vi "ADAM_Hi-Tec_convert.vi"(0 "Ch Name":string, 1 "Raw":dbl format="%.3f", 3 "Channel Read":string) -> (5 "Q release (l/min)":dbl format="%.2f", 6 "M_dot (kg/min)":dbl format="%.4f", 7 "Comments":string)   [LabVIEW 2022 SP3]
uses:
  Anemometry/Anemometry Sub Vis/Globals/Gas_management_global.vi
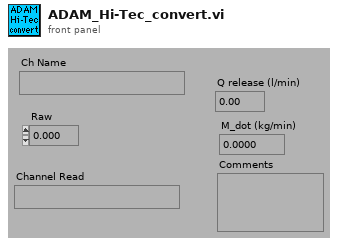
[diagram p1: front panel]
types:
  T1 = enum16{"Q(release) to Volts", "Volts to Q(release)"}
  T2 = typedef "Hi-Tec_calib.ctl" = cluster{"Ref temp (deg C)":dbl, "Ref Pres (mbars)":dbl, "Density at calib conditions":dbl, "Coefficients":dbl[], "Fit":T3}
  T3 = typedef "Hi-Tec Fitting.ctl" = enum16{"Polynomial", "Cubic Hermite Spline"}
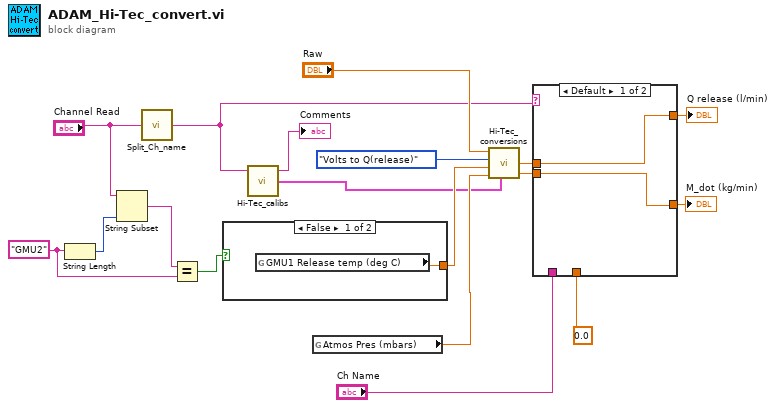
[diagram p0: block diagram]
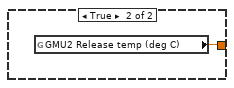
[diagram p2: hidden frame]
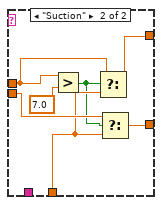
[diagram p3: hidden frame]
diagram:
  w2 = "GMU2"
  n1 = String Length(string=w2) -> (length=w5:i32)
  n2 = String Subset(string="Channel Read", length (rest)=w5) -> (substring=w3:string)  [unwired: 1 in]
  n3 = call "Split_Ch_name.vi"("Ch name"="Channel Read") -> ("Middle"=w8:string)  [unwired: 2 out]
  n4 = Equal?(x=w3, y=w2) -> (x = y?=w1:bool)
  n5 = case shown="False" w1 {
    tunnel: [w19 w20] -> w17
    frame False {
      n6 = global read "Gas_management_global.vi" "GMU1 Release temp (deg C)"() -> (w19:dbl)
    }
    frame True {
      n7 = global read "Gas_management_global.vi" "GMU2 Release temp (deg C)"() -> (w20:dbl)
    }
  }
  n8 = call "Hi-Tec_calibs.vi"("Gas Line Name"=w8) -> ("Hi-Tec calib"=w10:T2, "Comments"=→"Comments":string)  [unwired: 3 out]
  n9 = global read "Gas_management_global.vi" "Atmos Pres (mbars)"() -> (w16:dbl)
  n10 = call "Hi-Tec_conversions.vi"("Input"="Raw", "Conversion"=T1."Volts to Q(release)", "Release temp (deg C)"=w17, "Atmos Pres (mbars)"=w16, "Hi-Tec calib"=w10) -> ("Output"=w14:dbl, "Flowrate (kg/min)"=w12:dbl)  [unwired: 1 out]
  n11 = case shown="Default" w8 {
    tunnel: w14 -> [w22 w25]
    tunnel: [w22 w29] -> w13
    tunnel: w12 -> [w21 w28]
    tunnel: [w21 w27] -> w11
    tunnel: 0.0 -> [_ w26]
    tunnel: "Ch Name" -> [_ _]
    frame Default {
    }
    frame "Suction" {
      n12 = Greater?(x=w25, y=7.0) -> (0:w24:bool)
      n13 = Select(t=w25, s=w24, f=w26) -> (s? t:f=w29:dbl)
      n14 = Select(t=w28, s=w24, f=w26) -> (s? t:f=w27:dbl)
    }
  }
  "Q release (l/min)" <- w13
  "M_dot (kg/min)" <- w11
